vi "get UI reference.vi"(8 "error in":errorcluster, 11 "control label adjustment in":refnum<class "control label adjustment.lvclass">) -> (0 "error out":errorcluster, 2 "VI Refnum":refnum<vi>, 3 "control label adjustment out":refnum<class "control label adjustment.lvclass">)   [LabVIEW 2013, in "control label adjustment.lvclass"]
uses:
  control label adjustment.lvclass
  ctrl ui.vi
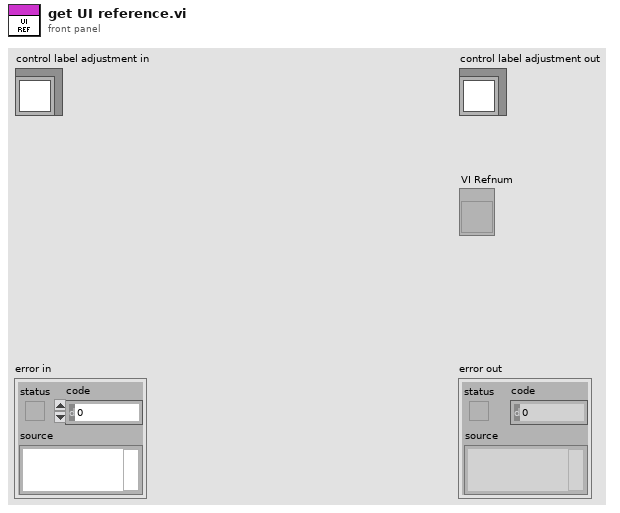
[diagram p1: front panel]
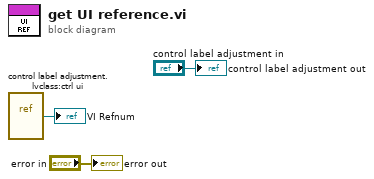
[diagram p0: block diagram]
diagram:
  n1 = vi-ref "control label adjustment.lvclass:ctrl ui.vi"() -> (→"VI Refnum":refnum<vi>)
  "error out" <- "error in"
  "control label adjustment out" <- "control label adjustment in"
